vi "Marshal.vi"(8 "error in (no error)":errorcluster, 11 "int32 in":refnum<class "float.lvclass">) -> (0 "error out":errorcluster, 2 "Buffer":u8[](array[numeric]), 3 "int32 out":refnum<class "float.lvclass">)   [LabVIEW 2020, in "Protobuf RAW.lvlib" / "float.lvclass"]
uses:
  float.lvclass
  float.lvclass/float.ctl
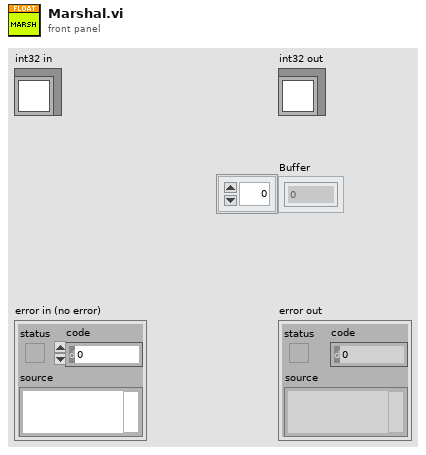
[diagram p1: front panel]
types:
  T1 = enum16{"big-endian, network order", "native, host order", "little-endian"}
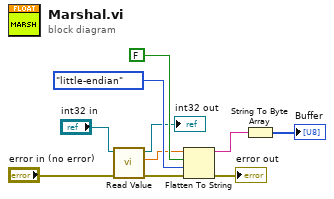
[diagram p0: block diagram]
diagram:
  n1 = call "Read Value.vi"("error in (no error)"="error in (no error)", "float in"="int32 in") -> ("error out"=w4:errorcluster, "Value"=w1:sgl, "float out"=→"int32 out":refnum<class "float.lvclass">)  [unwired: 7 in]
  n2 = Flatten To String(anything=w1, prepend array or string size? (T)=FALSE, byte order (0:big-endian, network order)=T1."little-endian", error in (no error)=w4) -> (data string=w7:string, error out=→"error out":errorcluster)  [unwired: 1 out]
  n3 = String To Byte Array(string=w7) -> (unsigned byte array=→"Buffer":u8[])
